vi "Engine Out - Faults - Oil Level Switch.vi"(11 "Oil Level [OFF=OK]":bool) -> ()   [LabVIEW 2015, in "ECS-RT.lvlib"]
uses:
  ECS-RT.lvlib
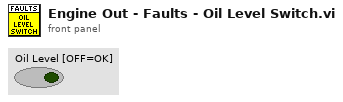
[diagram p1: front panel]
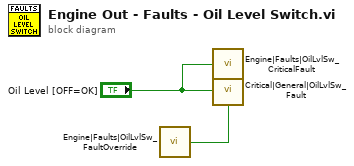
[diagram p0: block diagram]
diagram:
  n1 = call "Engine|Faults|OilLvlSw_FaultOverride"() -> ("Value"=w1:bool)
  n2 = call "Engine|Faults|OilLvlSw_CriticalFault"("Value"="Oil Level [OFF=OK]") -> ()
  n3 = call "Critical|General|OilLvlSw_Fault"("Fault"="Oil Level [OFF=OK]", "Override (F)"=w1) -> ()  [unwired: 1 in]
